vi "get_device_info.vi"(8 "error in (no error)":errorcluster caption="错误输入（无错误）", 11 "StepMotor输入":refnum<class "StepMotor.lvclass">) -> (0 "error out":errorcluster caption="错误输出", 2 "设备信息":T1, 3 "StepMotor输出":refnum<class "StepMotor.lvclass">)   [LabVIEW 2016, in "MotionControl_UFO_3DOF.lvlib" / "StepMotor.lvclass"]
uses:
  <userlib>/MotionControl_UFO_3DOF/StepMotor/StepMotor.lvclass
  <userlib>/MotionControl_UFO_3DOF/StepMotor/StepMotor.lvclass/StepMotor.ctl
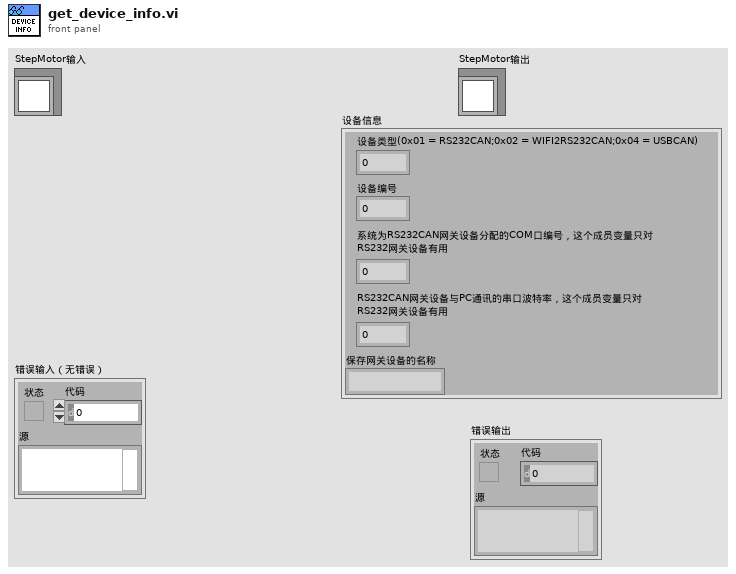
[diagram p1: front panel]
types:
  T1 = cluster{"设备类型(0x01 = RS232CAN;0x02 = WIFI2RS232CAN;0x04 = USBCAN)":u32, "设备编号":u32, "系统为RS232CAN网关设备分配的COM口编号，这个成员变量只对\nRS232网关设备有用":u32, "RS232CAN网关设备与PC通讯的串口波特率，这个成员变量只对\nRS232网关设备有用":u32, "保存网关设备的名称":string}
  T2 = typedef "MotionControl_UFO_3DOF.lvlib/StepMotor.lvclass/DEV_INFO.ctl" = cluster{"设备类型(0x01 = RS232CAN;0x02 = WIFI2RS232CAN;0x04 = USBCAN)":u32, "设备编号":u32, "系统为RS232CAN网关设备分配的COM口编号，这个成员变量只对\nRS232网关设备有用":u32, "RS232CAN网关设备与PC通讯的串口波特率，这个成员变量只对\nRS232网关设备有用":u32, "保存网关设备的名称":string}
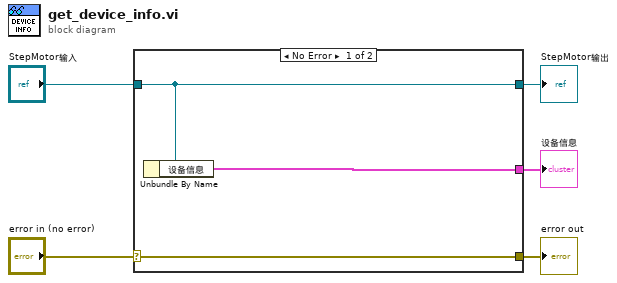
[diagram p0: block diagram]
diagram:
  n1 = case shown="No Error" "error in (no error)" {
    selector: "error in (no error)" -> [w8 w9]
    tunnel: [w8 w9] -> w4
    tunnel: [w7 w10] -> w2
    tunnel: "StepMotor输入" -> [w7 w10]
    tunnel: [w6 _] -> w1
    frame No Error {
      n2 = Unbundle By Name(w7) -> ("设备信息"=w6:T2)
    }
    frame Error {
    }
  }
  "error out" <- w4
  "StepMotor输出" <- w2
  "设备信息" <- w1
